vi "正则match_numbers.vi"() -> ()   [LabVIEW 2022 SP3]
panel:
  out "results":string[](array[string])
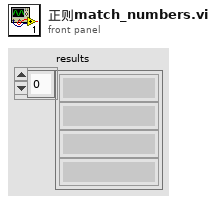
[diagram p1: front panel]
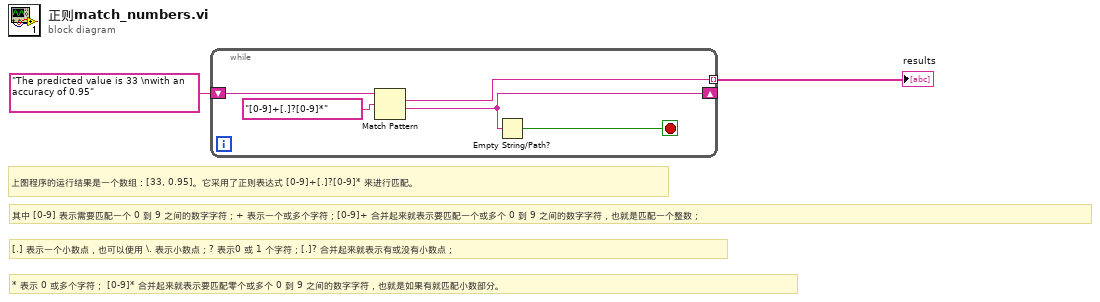
[diagram p0: block diagram]
diagram:
  # "* 表示 0 或多个字符； [0-9]* 合并起来就表示要匹配零个或多个 0 到 9 之间的数字字符，也就是如果有就匹配小数部分。"
  # "[.] 表示一个小数点，也可以使用 \\. 表示小数点；? 表示0 或 1 个字符；[.]? 合并起来就表示有或没有小数点；"
  # "其中 [0-9] 表示需要匹配一个 0 到 9 之间的数字字符；+ 表示一个或多个字符；[0-9]+ 合并起来就表示要匹配一个或多个 0 到 9 之间的数字字符，也就是匹配一个整数；"
  # "上图程序的运行结果是一个数组：[33, 0.95]。它采用了正则表达式 [0-9]+[.]?[0-9]* 来进行匹配。"
  n1 = while {
    shift-right: [w4] -> _
    shift-left: "The predicted value is 33 \nwith an accuracy of 0.95" -> [w7]
    tunnel: [w5] -> w1 mode=indexing
    stop <- w3 stop-if-true
    n2 = Match Pattern(string=w7, regular expression="[0-9]+[.]?[0-9]*") -> (match substring=w5:string, after substring=w4:string)  [unwired: 1 in, 2 out]
    n3 = Empty String/Path?(string/path=w4) -> (empty?=w3:bool)
  }
  "results" <- w1
